vi "PXIe-4139 Get Channel Indices (RT).vi"(8 "error in (no error)":errorcluster, 11 "Device Item Ref In":T1 format="%.0x") -> (0 "error out":errorcluster, 1 "Read Trigger Index":i32, 2 "Continuous Read? Index":i32, 3 "Device Item Ref Out":T1 format="%.0x", 5 "error index":i32, 7 "channel output FIFO indexes":i32[](array[numeric]))   [LabVIEW 2023, in "PXIe-4139 Custom Device.lvlib"]
uses:
  PXIe-4139 Custom Device.lvlib
  <vilib>/NI VeriStand/Custom Device API/Custom Device Item Ref.ctl
  PXIe-4139 Global Variable.vi
  <vilib>/NI VeriStand/Custom Device Tools/Custom Device Utility Library/NI VeriStand - Search for Item by GUID.vi
  <vilib>/NI VeriStand/Custom Device Tools/Custom Device Utility Library/Custom Device Utility Library.lvlib
  <vilib>/NI VeriStand/Custom Device API/Custom Device API.lvlib
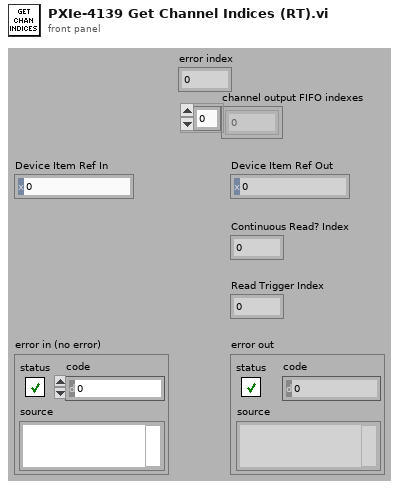
[diagram p1: front panel]
types:
  T1 = typedef "Custom Device API.lvlib/Custom Device Item Ref.ctl" = u64
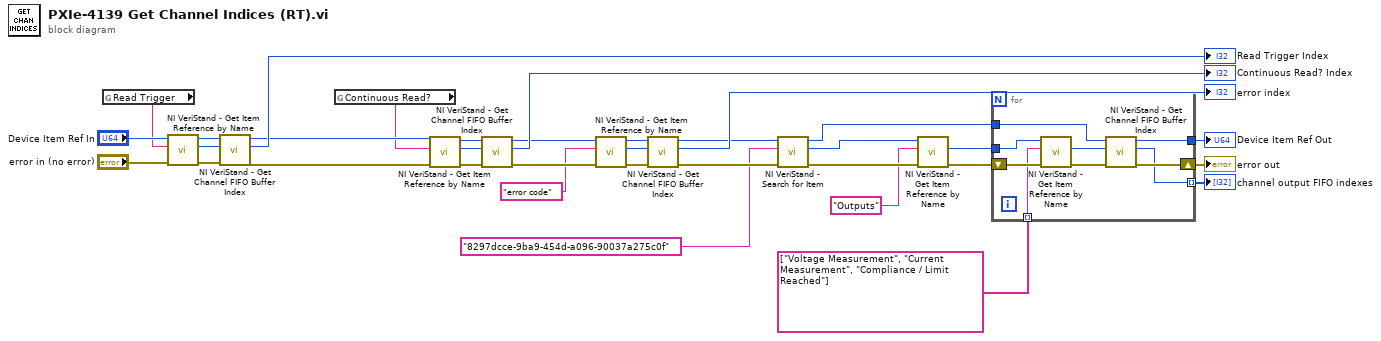
[diagram p0: block diagram]
diagram:
  n1 = global read "PXIe-4139 Global Variable.vi" "Read Trigger"() -> (w30:string)
  n2 = call <vilib>:"NI VeriStand - Get Item Reference by Name.vi"("error in (no error)"="error in (no error)", "Item Name"=w30, "Parent Ref in"="Device Item Ref In") -> ("error out"=w28:errorcluster, "Item Ref"=w31:T1, "Parent Ref out"=w32:T1)  [unwired: 5 in, 1 out]
  n3 = call <vilib>:"NI VeriStand - Get Channel FIFO Buffer Index.vi"("error in"=w28, "Channel Ref"=w31, "Device Ref in"=w32) -> ("error out"=w23:errorcluster, "Channel FIFO Buffer Index"=→"Read Trigger Index":i32, "Device Ref out"=w24:T1)  [unwired: 4 in, 2 out]
  n4 = global read "PXIe-4139 Global Variable.vi" "Continuous Read?"() -> (w22:string)
  n5 = call <vilib>:"NI VeriStand - Get Item Reference by Name.vi"("error in (no error)"=w23, "Item Name"=w22, "Parent Ref in"=w24) -> ("error out"=w27:errorcluster, "Item Ref"=w26:T1, "Parent Ref out"=w25:T1)  [unwired: 5 in, 1 out]
  n6 = call <vilib>:"NI VeriStand - Get Channel FIFO Buffer Index.vi"("error in"=w27, "Channel Ref"=w26, "Device Ref in"=w25) -> ("error out"=w19:errorcluster, "Channel FIFO Buffer Index"=→"Continuous Read? Index":i32, "Device Ref out"=w18:T1)  [unwired: 4 in, 2 out]
  n7 = call <vilib>:"NI VeriStand - Get Item Reference by Name.vi"("error in (no error)"=w19, "Item Name"="error code", "Parent Ref in"=w18) -> ("error out"=w20:errorcluster, "Item Ref"=w2:T1, "Parent Ref out"=w1:T1)  [unwired: 5 in, 1 out]
  n8 = call <vilib>:"NI VeriStand - Get Channel FIFO Buffer Index.vi"("error in"=w20, "Channel Ref"=w2, "Device Ref in"=w1) -> ("error out"=w16:errorcluster, "Channel FIFO Buffer Index"=→"error index":i32, "Device Ref out"=w14:T1)  [unwired: 4 in, 2 out]
  n9 = call-poly <vilib>:"NI VeriStand - Search for Item.vi"("error in"=w16, "Item GUID"="8297dcce-9ba9-454d-a096-90037a275c0f", "Section Ref in"=w14) -> ("error out"=w12:errorcluster, "Item Ref"=w11:T1, "Section Ref out"=w6:T1)  [unwired: 5 in, 1 out]
  n10 = call <vilib>:"NI VeriStand - Get Item Reference by Name.vi"("error in (no error)"=w12, "Item Name"="Outputs" ("Section Name"), "Parent Ref in"=w11) -> ("error out"=w9:errorcluster, "Item Ref"=w8:T1)  [unwired: 5 in, 2 out]
  n11 = for {
    shift-right: [w37] -> w4
    shift-left: w9 -> [w43]
    tunnel: w8 -> [w42]
    tunnel: string[] ["Voltage Measurement", "Current Measurement", "Compliance / Limit Reached"] -> [w41] mode=indexing
    tunnel: w6 -> [w38]
    tunnel: [w36] -> w5
    tunnel: [w35] -> w3 mode=indexing
    n12 = call <vilib>:"NI VeriStand - Get Item Reference by Name.vi"("error in (no error)"=w43, "Item Name"=w41, "Parent Ref in"=w42) -> ("error out"=w40:errorcluster, "Item Ref"=w39:T1)  [unwired: 5 in, 2 out]
    n13 = call <vilib>:"NI VeriStand - Get Channel FIFO Buffer Index.vi"("error in"=w40, "Channel Ref"=w39, "Device Ref in"=w38) -> ("error out"=w37:errorcluster, "Channel FIFO Buffer Index"=w35:i32, "Device Ref out"=w36:T1)  [unwired: 4 in, 2 out]
  }
  "Device Item Ref Out" <- w5
  "error out" <- w4
  "channel output FIFO indexes" <- w3
